vi "Validate Checksum.vi"(11 "Buffer":u8[](array[numeric])) -> (3 "Checksum Valid?":bool)   [LabVIEW 2010]
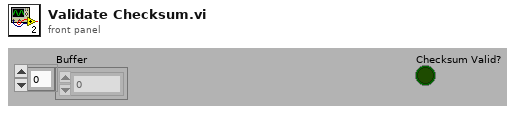
[diagram p1: front panel]
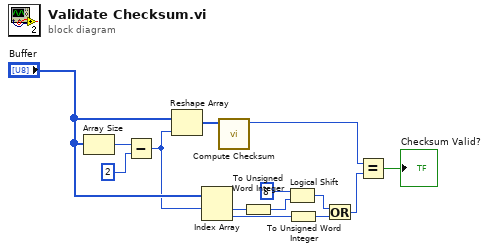
[diagram p0: block diagram]
diagram:
  n1 = Array Size(array="Buffer") -> (size(s)=w14:i32)
  n2 = Subtract(x=w14, y=2 ("x")) -> (x-y=w1:i32)
  n3 = Reshape Array("Buffer", w1) -> (w12:u8[])
  n4 = Index Array(array="Buffer", index #1=w1) -> (element #1=w8:u8, element #2=w6:u8)  [unwired: 1 in]
  n5 = call "Compute Checksum.vi"("Command"=w12) -> ("Checksum"=w4:u16)  [unwired: 10 in]
  n6 = To Unsigned Word Integer(number=w8) -> (unsigned 16bit integer=w7:u16)
  n7 = Logical Shift(y=i16 8, x=w7) -> (x << y=w9:u16)
  n8 = To Unsigned Word Integer(number=w6) -> (unsigned 16bit integer=w5:u16)
  n9 = Or(x=w9, y=w5) -> (x .or. y?=w3:u16)
  n10 = Equal?(x=w4, y=w3) -> (x = y?=→"Checksum Valid?":bool)
